vi "Move to next loop.vi"(9 "Fwd (T): Rev (F)":bool, 10 "Position in":cluster{i32, i32}, 11 "Map in":T1(c390)) -> (1 "Start?":bool, 2 "Position out":cluster{i32, i32}, 3 "Map out":T1(c390))   [LabVIEW 2023, in "d10.lvlib"]
uses:
  d10.lvlib
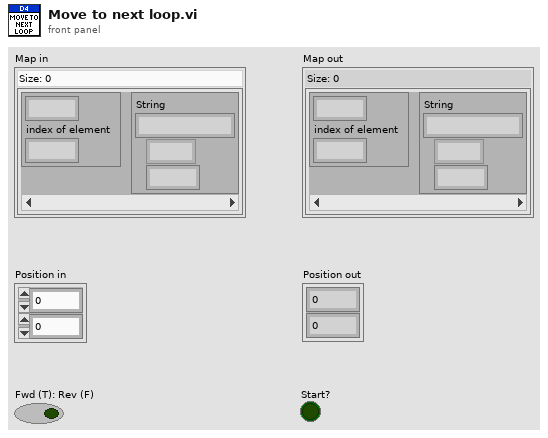
[diagram p1: front panel]
types:
  T1 = map{cluster{i32, "index of element":i32}, cluster{"String":string, enum16{"unvisited", "loop", "in", "out"}, u64}}
  T2 = cluster{"String":string, enum16{"unvisited", "loop", "in", "out"}, u64}
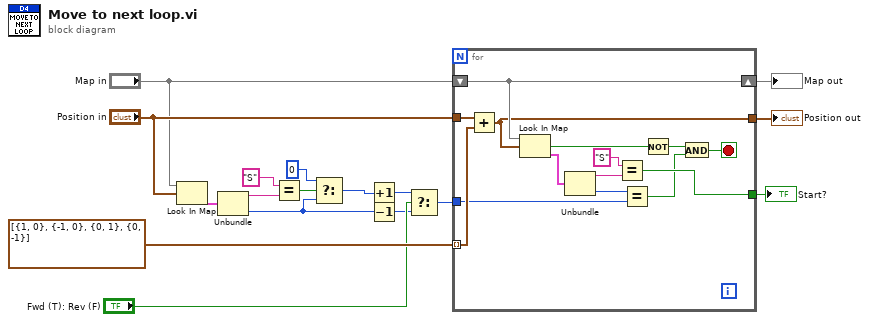
[diagram p0: block diagram]
diagram:
  n1 = Look In Map(map="Map in", key="Position in") -> (value=w11:T2)  [unwired: 1 in, 1 out]
  n2 = Unbundle(w11) -> ("String"=w6:string, w2:u64)  [unwired: 1 out]
  n3 = Equal?(x="S" ("y"), y=w6) -> (x = y?=w4:bool)
  n4 = Select(t=u64 0, s=w4, f=w2) -> (s? t:f=w1:u64)
  n5 = Increment(x=w1) -> (x+1=w9:u64)
  n6 = Decrement(x=w2) -> (x-1=w7:u64)
  n7 = Select(t=w9, s="Fwd (T): Rev (F)", f=w7) -> (s? t:f=w8:u64)
  n8 = for {
    tunnel: cluster{i32, i32}[] [{1, 0}, {-1, 0}, {0, 1}, {0, -1}] -> [w30] mode=indexing
    tunnel: "Position in" -> [w31]
    shift-right: [w29] -> w17
    shift-left: "Map in" -> [w29]
    tunnel: [w25] -> w16
    tunnel: [w21] -> w12
    tunnel: w8 -> [w19]
    stop <- w24 stop-if-true
    n9 = Add(x=w31, y=w30) -> (x+y=w25:cluster{i32, i32})
    n10 = Look In Map(map=w29, key=w25) -> (key not found?=w28:bool, value=w27:T2)  [unwired: 1 in]
    n11 = Unbundle(w27) -> ("String"=w22:string, w20:u64)  [unwired: 1 out]
    n12 = Equal?(x="S" ("y"), y=w22) -> (x = y?=w21:bool)
    n13 = Equal?(x=w20, y=w19) -> (x = y?=w18:bool)
    n14 = Not(x=w28) -> (.not. x?=w26:bool)
    n15 = And(x=w26, y=w18) -> (x .and. y?=w24:bool)
  }
  "Position out" <- w16
  "Map out" <- w17
  "Start?" <- w12
